vi "writeToXML.vi"(8 "error in (no error)":errorcluster, 10 "Class Label":string="RADecParameters", 11 "RADecParameters in":refnum<class "RADecParameters.lvclass">) -> (0 "error out":errorcluster, 2 "XML out":string, 3 "RADecParameters out":refnum<class "RADecParameters.lvclass">)   [LabVIEW 2014, in "TCSDataDefinitions.lvlib" / "TCSCommand.lvlib" / "TargetConfiguration.lvlib" / "Target.lvlib" / "FixedTarget.lvlib" / "RADecParameters.lvclass"]
uses:
  RADecParameters.lvclass
  RADecParameters.lvclass/RADecParameters.ctl
  Declination/Declination.lvclass
  TCSPublicStatus/CurrentTimes/ClockTimes/ClockTimes.lvclass
  <userlib>/Common/XML/XMLGenerator/XMLGenerator.lvclass
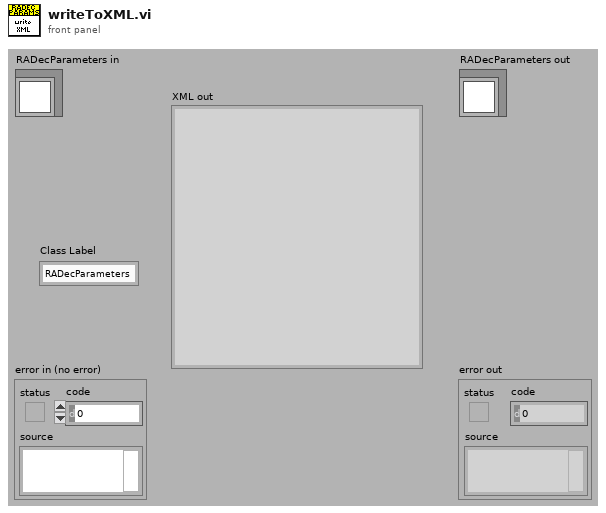
[diagram p1: front panel]
types:
  T1 = typedef "TCSDataDefinitions.lvlib/TCSCommand.lvlib/TargetConfiguration.lvlib/Target.lvlib/FixedTarget.lvlib/EquinoxPrefix.ctl" = enum16{"B", "J"}
  T2 = typedef "TCSDataDefinitions.lvlib/TCSCommand.lvlib/TargetConfiguration.lvlib/Target.lvlib/FixedTarget.lvlib/FrameValues.ctl" = enum16{"FK4", "FK5", "APPT", "GAPPT", "AZEL"}
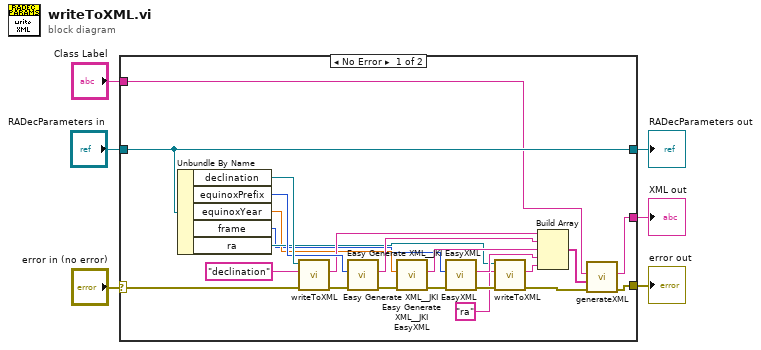
[diagram p0: block diagram]
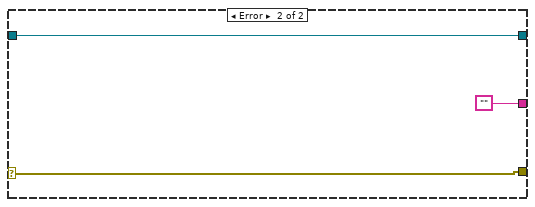
[diagram p2: hidden frame]
diagram:
  n1 = case shown="No Error" "error in (no error)" {
    selector: "error in (no error)" -> [w26 w32]
    tunnel: [w17 w32] -> w5
    tunnel: [w23 w31] -> w3
    tunnel: "RADecParameters in" -> [w23 w31]
    tunnel: "Class Label" -> [w7 _]
    tunnel: [w8 ""] -> w1
    frame No Error {
      n2 = Unbundle By Name(w23) -> ("declination"=w29:refnum<class "Declination.lvclass">, "equinoxPrefix"=w28:T1, "equinoxYear"=w10:dbl, "frame"=w9:T2, "ra"=w11:refnum<class "ClockTimes.lvclass">)
      n3 = call-dynamic "writeToXML.vi"("error in (no error)"=w26, "Class Label"="declination", "Declination in"=w29) -> ("error out"=w27:errorcluster, "XML out"=w24:string)  [unwired: 6 in, 1 out]
      n4 = call <vilib>:"Easy Generate XML__JKI EasyXML.vi"("error in (no error)"=w27, "LabVIEW Data"=w28) -> ("error out"=w21:errorcluster, "XML String"=w22:string)  [unwired: 8 in]
      n5 = call <vilib>:"Easy Generate XML__JKI EasyXML.vi"("error in (no error)"=w21, "LabVIEW Data"=w10) -> ("error out"=w20:errorcluster, "XML String"=w15:string)  [unwired: 8 in]
      n6 = call <vilib>:"Easy Generate XML__JKI EasyXML.vi"("error in (no error)"=w20, "LabVIEW Data"=w9) -> ("error out"=w19:errorcluster, "XML String"=w14:string)  [unwired: 8 in]
      n7 = call-dynamic "writeToXML.vi"("error in (no error)"=w19, "Class Label"="ra", "ClockTimes in"=w11) -> ("error out"=w18:errorcluster, "XML out"=w13:string)  [unwired: 6 in, 1 out]
      n8 = Build Array(w24, w22, w15, w14, w13) -> (w16:string[])
      n9 = call <userlib>:"generateXML.vi"("error in"=w18, "childrenXML"=w16, "elementName"=w7) -> ("error out"=w17:errorcluster, "XML out"=w8:string)  [unwired: 6 in, 1 out]
    }
    frame Error {
    }
  }
  "error out" <- w5
  "RADecParameters out" <- w3
  "XML out" <- w1
